vi "Send Monitor Stop.vi"(7 "Priority":T2 caption="Message Priority (Normal)", 8 "error in (no error)":errorcluster, 10 "Actor Data":T1={"Actor Type"="", "Actor Cores"=[], "Self"=refnum, "Caller"=refnum, "Actor Label"="", "Last Ping"=-1.0}, 11 "Message Enqueuer in":refnum<class "Message Enqueuer.lvclass">) -> (0 "error out":errorcluster, 3 "Message Enqueuer out":refnum<class "Message Enqueuer.lvclass">)   [LabVIEW 2017, in "MGI-Monitored Actor.lvlib" / "Monitor Stop Msg.lvclass"]
doc: "Sends the <b>Monitored Actor.lvlib:Monitor Stop Msg.lvclass</b> message.\n\nThis message will call <b>Monitor Stop.vi</b> on the <b>Monitored Actor.lvlib:Orphan Detector.lvclass</b> actor.\n\n<b>Monitor Stop.vi Description</b>"
uses:
  Monitor Stop Msg.lvclass
  <vilib>/ActorFramework/Message Enqueuer/Message Enqueuer.lvclass
  <vilib>/ActorFramework/Message Enqueuer/Message Priority.ctl
  monitored-actor-core/Source/Monitor Data/Actor Data.ctl
  C:/Program Files (x86)/National Instruments/LabVIEW 2017/vi.lib/ActorFramework/Message/Message.lvclass
  Monitor Stop Msg.lvclass/Monitor Stop Msg.ctl
  <vilib>/ActorFramework/Message Enqueuer/Message Enqueuer.lvclass/Message Enqueuer.ctl
  <vilib>/ActorFramework/Message Priority Queue/Priority Enqueue.vi
  monitored-actor-core/Source/Monitor Data/Monitor Data.lvclass
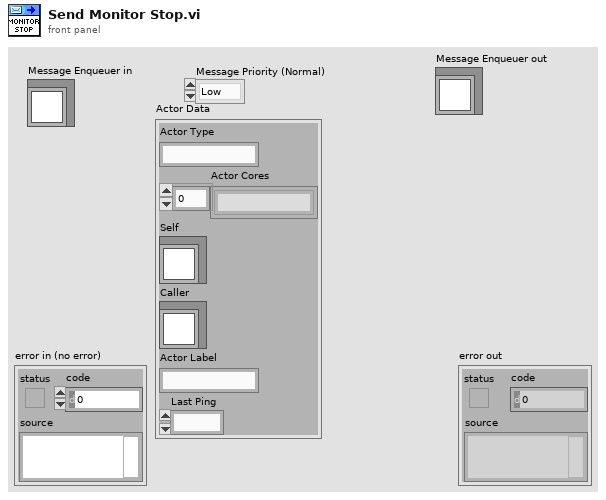
[diagram p1: front panel]
types:
  T1 = typedef "MGI-Monitored Actor Core.lvlib/Monitor Data.lvclass/Actor Data.ctl" = cluster{"Actor Type":string, "Actor Cores":string[], "Self":refnum<class "Message Enqueuer.lvclass">, "Caller":refnum<class "Message Enqueuer.lvclass">, "Actor Label":string, "Last Ping":dbl}
  T2 = typedef "Actor Framework.lvlib/Message Enqueuer.lvclass/Message Priority.ctl" = enum16{"Low", "Normal", "High"}
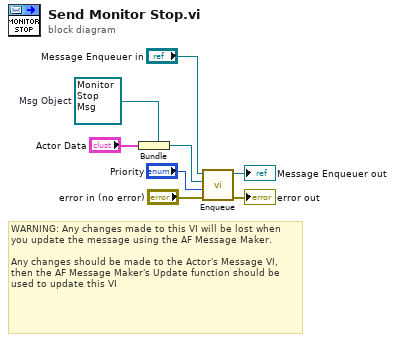
[diagram p0: block diagram]
diagram:
  w7 = refnum<class "Monitor Stop Msg.lvclass"> refnum  # Msg Object
  # "WARNING: Any changes made to this VI will be lost when you update the message using the AF Message Maker.\n\nAny changes should be made to the Actor's Message VI, then the AF Message Maker's Update function should be used to update this VI"
  n1 = Bundle(cluster=w7, "Actor Data") -> (w2:refnum<class "Monitor Stop Msg.lvclass">)
  n2 = call <vilib>:"Enqueue.vi"("error in (no error)"="error in (no error)", "Message Priority (Normal)"="Priority", "Message"=w2, "Message Enqueuer in"="Message Enqueuer in") -> ("error out"=→"error out":errorcluster, "Message Enqueuer out"=→"Message Enqueuer out":refnum<class "Message Enqueuer.lvclass">)  [unwired: 6 in]
